vi "Get Intensity Graph X Scale.vi"(8 "error in (no error)":errorcluster, 11 "graph_utilities in":refnum<class "graph_utilities.lvclass">) -> (0 "error out":errorcluster, 1 "X Scale.Offset and Multiplier":T1, 2 "X Scale":dbl[](array[numeric]), 3 "graph_utilities out":refnum<class "graph_utilities.lvclass">)   [LabVIEW 2016, in "graph_utilities.lvclass"]
doc: "Get the X Scale of the Intensity Graph (Both X Array and X Offset and Multiplier)"
uses:
  graph_utilities.lvclass
  <vilib>/Utility/miscctls.llb/LVOffsetAndMultiplierTypeDef.ctl
  graph_utilities.lvclass/graph_utilities.ctl
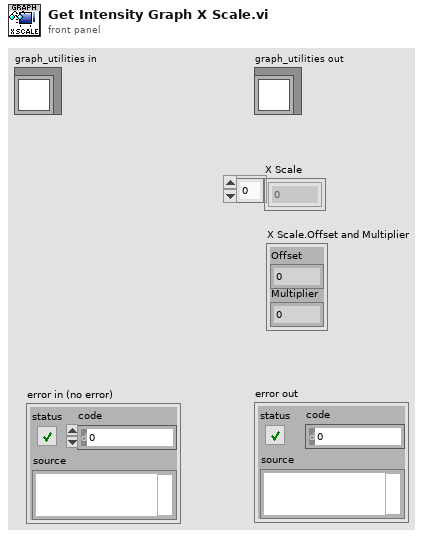
[diagram p1: front panel]
types:
  T1 = typedef "LVOffsetAndMultiplierTypeDef.ctl" = cluster{"Offset":dbl, "Multiplier":dbl}
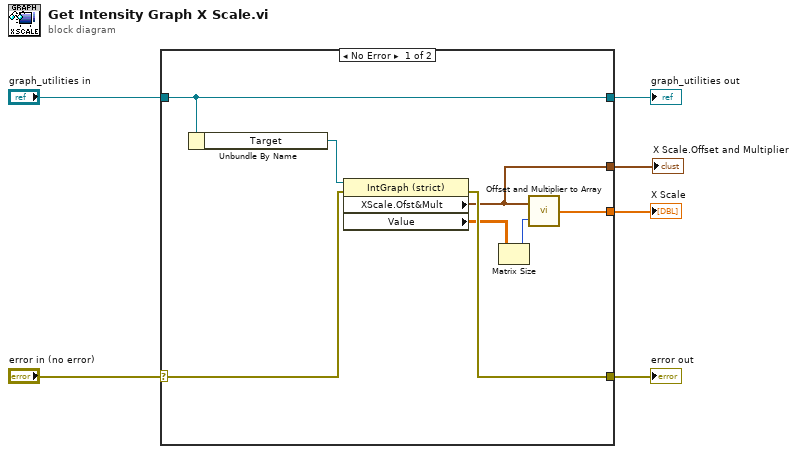
[diagram p0: block diagram]
diagram:
  n1 = case shown="No Error" "error in (no error)" {
    selector: "error in (no error)" -> [w11 w16]
    tunnel: [w14 w16] -> w6
    tunnel: "graph_utilities in" -> [w13 w15]
    tunnel: [w13 w15] -> w3
    tunnel: [w8 _] -> w2
    tunnel: [w7 _] -> w1
    frame No Error {
      n2 = Unbundle By Name(w13) -> ("Target"=w12:refnum<vi>)
      n3 = property on="Property Node" class="IntGraph (strict)"(reference=w12, error in=w11) -> (error out=w14:errorcluster, "XScale.Ofst&Mult"=w7:T1, "Value"=w10:dbl[][])  [unwired: 1 out]
      n4 = Matrix Size(0:w10) -> (1:w9:i32)  [unwired: 1 out]
      n5 = call "Offset and Multiplier to Array.vi"("Size"=w9, "Offset and Multiplier"=w7) -> ("Array"=w8:dbl[])
    }
    frame Error {
    }
  }
  "X Scale" <- w2
  "error out" <- w6
  "graph_utilities out" <- w3
  "X Scale.Offset and Multiplier" <- w1
